vi "Cobalt532.vi"(1 "error in":errorcluster, 2 "command":string) -> (0 "error out":errorcluster)   [LabVIEW 2013]
uses:
  <vilib>/DAQmx/write.llb/DAQmx Write (Digital Bool 1Line 1Point).vi
  <vilib>/DAQmx/create/channels.llb/DAQmx Create Channel (DO-Digital Output).vi
  <vilib>/DAQmx/miscellaneous.llb/DAQmx Fill In Error Info.vi
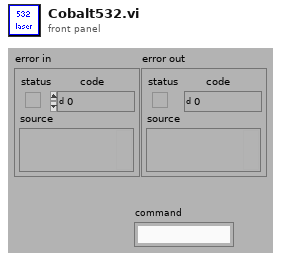
[diagram p1: front panel]
types:
  T1 = cluster{"CH1 AI":tag, "CH1 CI":tag, "CH2 AI":tag, "CH2 CI":tag, "AI X":tag, "AI Y":tag, "AO X-Y":tag, "CH1ST":bool, "CH2ST":bool, "Sigcase":i16, "StageS":i32, "StageL":i32, "data dir":path, "AI VC":tag, "AI CC":tag, "AO CWlaser":tag, "AO VtoP":tag, "shutter":tag, "488":tag, "532":tag, "640":tag}
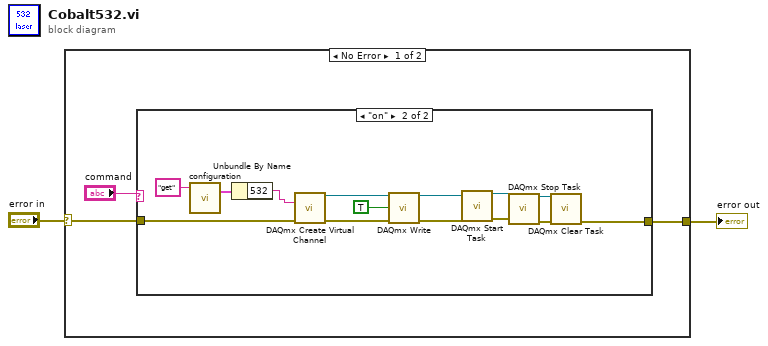
[diagram p0: block diagram]
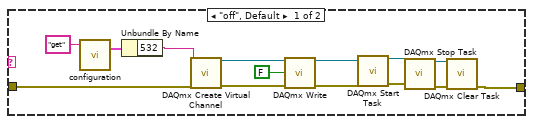
[diagram p2: hidden frame]
diagram:
  n1 = case shown="No Error" "error in" {
    selector: "error in" -> [w4 w34]
    tunnel: [w3 w34] -> w1
    frame No Error {
      n2 = case shown="\"on\"" "command" {
        tunnel: w4 -> [w10 w25]
        tunnel: [w9 w24] -> w3
        frame "off", Default {
          n3 = call "configuration.vi"("command"="get") -> ("config out"=w8:T1)  [unwired: 2 in, 1 out]
          n4 = Unbundle By Name(w8) -> ("532"=w6:tag)
          n5 = call-poly <vilib>:"DAQmx Create Virtual Channel.vi"("lines"=w6, "error in"=w10) -> ("task out"=w13:refnum<k21>, "error out"=w12:errorcluster)  [unwired: 12 in]
          n6 = call-poly <vilib>:"DAQmx Write.vi"("task/channels in"=w13, "data"=FALSE, "error in"=w12) -> ("task out"=w14:refnum<k21>, "error out"=w15:errorcluster)  [unwired: 10 in, 1 out]
          n7 = call <vilib>:"DAQmx Start Task.vi"("task/channels in"=w14, "error in"=w15) -> ("task out"=w16:refnum<k21>, "error out"=w17:errorcluster)  [unwired: 12 in]
          n8 = call <vilib>:"DAQmx Stop Task.vi"("task/channels in"=w16, "error in"=w17) -> ("task out"=w18:refnum<k21>, "error out"=w19:errorcluster)  [unwired: 12 in]
          n9 = call <vilib>:"DAQmx Clear Task.vi"("task in"=w18, "error in"=w19) -> ("error out"=w9:errorcluster)  [unwired: 13 in]
        }
        frame "on" {
          n10 = call "configuration.vi"("command"="get") -> ("config out"=w22:T1)  [unwired: 2 in, 1 out]
          n11 = Unbundle By Name(w22) -> ("532"=w20:tag)
          n12 = call-poly <vilib>:"DAQmx Create Virtual Channel.vi"("lines"=w20, "error in"=w25) -> ("task out"=w27:refnum<k21>, "error out"=w26:errorcluster)  [unwired: 12 in]
          n13 = call-poly <vilib>:"DAQmx Write.vi"("task/channels in"=w27, "data"=TRUE, "error in"=w26) -> ("task out"=w28:refnum<k21>, "error out"=w29:errorcluster)  [unwired: 10 in, 1 out]
          n14 = call <vilib>:"DAQmx Start Task.vi"("task/channels in"=w28, "error in"=w29) -> ("task out"=w30:refnum<k21>, "error out"=w31:errorcluster)  [unwired: 12 in]
          n15 = call <vilib>:"DAQmx Stop Task.vi"("task/channels in"=w30, "error in"=w31) -> ("task out"=w32:refnum<k21>, "error out"=w33:errorcluster)  [unwired: 12 in]
          n16 = call <vilib>:"DAQmx Clear Task.vi"("task in"=w32, "error in"=w33) -> ("error out"=w24:errorcluster)  [unwired: 13 in]
        }
      }
    }
    frame Error {
    }
  }
  "error out" <- w1
